vi "Search Stop Module.vi"(11 "Child Tree":string="\\DQMH Modules\\Cloneable Module.lvlib\\Request") -> (3 "Stop Module path":string)   [LabVIEW 2020, in "Panther Dashboard.lvlib"]
uses:
  Panther Dashboard.lvlib
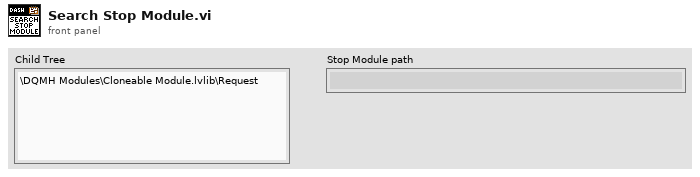
[diagram p1: front panel]
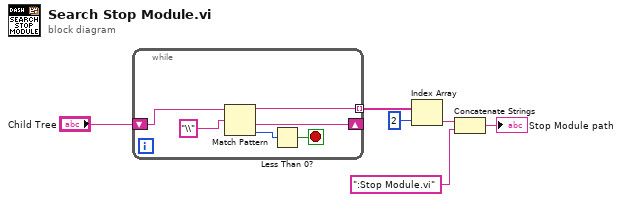
[diagram p0: block diagram]
diagram:
  n1 = while {
    shift-right: [w10] -> _
    shift-left: "Child Tree" -> [w12]
    tunnel: [w9] -> w5 mode=indexing
    stop <- w7 stop-if-true
    n2 = Match Pattern(string=w12, regular expression="\\") -> (before substring=w9:string, after substring=w10:string, offset past match=w8:i32)  [unwired: 1 in, 1 out]
    n3 = Less Than 0?(x=w8) -> (x < 0?=w7:bool)
  }
  n4 = Index Array(array=w5, index=2) -> (element=w3:string)
  n5 = Concatenate Strings(w3, ":Stop Module.vi" ("string")) -> (→"Stop Module path":string)
